vi "Get Tree Refnum.vi"(8 "error in (no error)":errorcluster, 11 "TREE in":refnum<class "MyTreeAPI.lvclass">) -> (0 "error out":errorcluster, 2 "Tree":refnum<vi>, 3 "TREE out":refnum<class "MyTreeAPI.lvclass">)   [LabVIEW 2015, in "MyTreeAPI.lvclass"]
uses:
  MyTreeAPI.lvclass
  MyTreeAPI.lvclass/MyTreeAPI.ctl
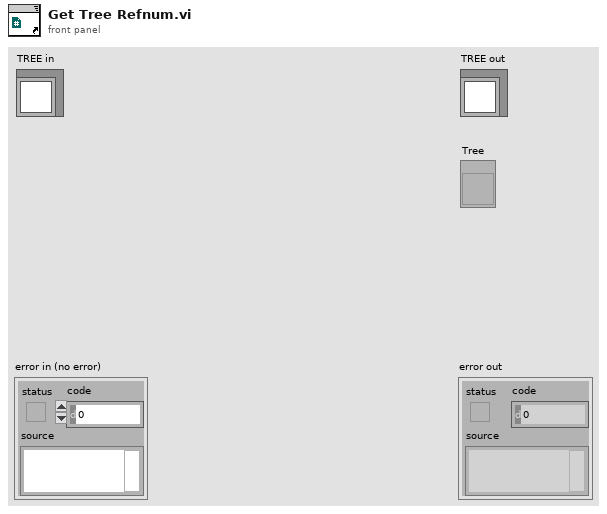
[diagram p1: front panel]
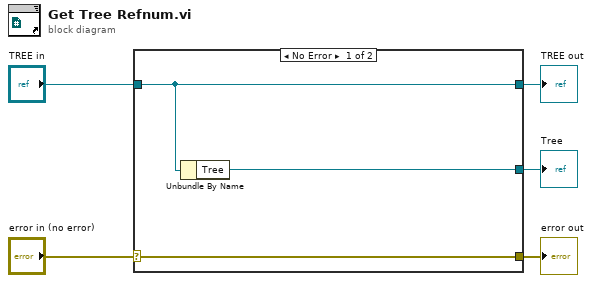
[diagram p0: block diagram]
diagram:
  n1 = case shown="No Error" "error in (no error)" {
    selector: "error in (no error)" -> [w8 w9]
    tunnel: [w8 w9] -> w4
    tunnel: [w7 w10] -> w2
    tunnel: "TREE in" -> [w7 w10]
    tunnel: [w6 _] -> w1
    frame No Error {
      n2 = Unbundle By Name(w7) -> ("Tree"=w6:refnum<vi>)
    }
    frame Error {
    }
  }
  "error out" <- w4
  "TREE out" <- w2
  "Tree" <- w1
